vi "题目1.vi"() -> ()   [LabVIEW 2017]
panel:
  out "元素 4":i32
  out "元素 3":i32
  out "元素 2":i32
  out "元素":i32
  out "数组":i32[](array[numeric])
  out "添加的数组":i32[](array[numeric])
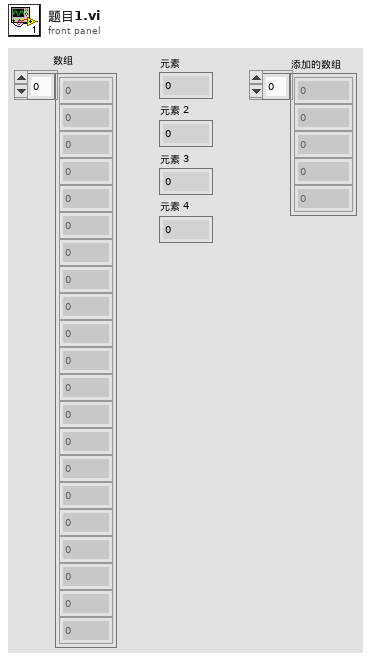
[diagram p1: front panel]
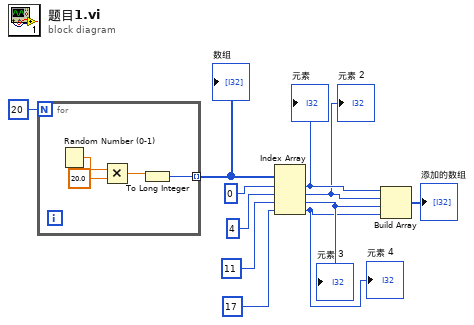
[diagram p0: block diagram]
diagram:
  n1 = for {
    N: 20 -> [_]
    tunnel: [w12] -> w9 mode=indexing
    n2 = Random Number (0-1)() -> (number: 0 to 1=w15:dbl)
    n3 = Multiply(x=w15, y=20.0) -> (x*y=w13:dbl)
    n4 = To Long Integer(number=w13) -> (32bit integer=w12:i32)
  }
  "数组" <- w9
  n5 = Index Array(array=w9, index #1=0 ("索引"), index #2=4 ("索引"), index #3=11 ("索引"), index #4=17 ("索引")) -> (element #1=w5:i32, element #2=w4:i32, element #3=w3:i32, element #4=w2:i32)
  "元素" <- w5
  "元素 2" <- w4
  "元素 3" <- w3
  "元素 4" <- w2
  n6 = Build Array(w5, w4, w3, w2) -> (→"添加的数组":i32[])
